vi "WriteAsyncErrorHandling.vi"(8 "ErrorIn":errorcluster, 10 "AsyncErrorHandling":T1, 11 "YActorIn":refnum<class "YActor.lvclass">) -> (0 "ErrorOut":errorcluster, 3 "YActorOut":refnum<class "YActor.lvclass">)   [LabVIEW 2021, in "YActor.lvclass"]
uses:
  YActor.lvclass
  AsyncErrorHandling.ctl
  YActor.lvclass/YActor.ctl
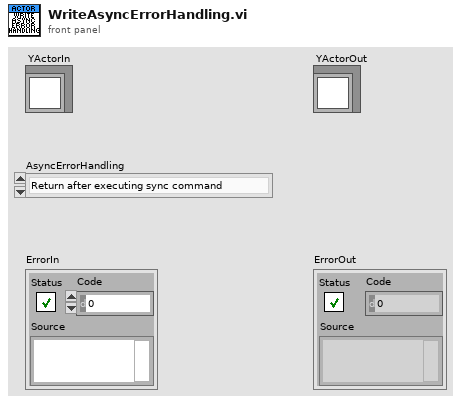
[diagram p1: front panel]
types:
  T1 = typedef "YActor.lvclass/AsyncErrorHandling.ctl" = enum16{"Return after executing sync command", "Return before executing sync command", "Don't return error"}
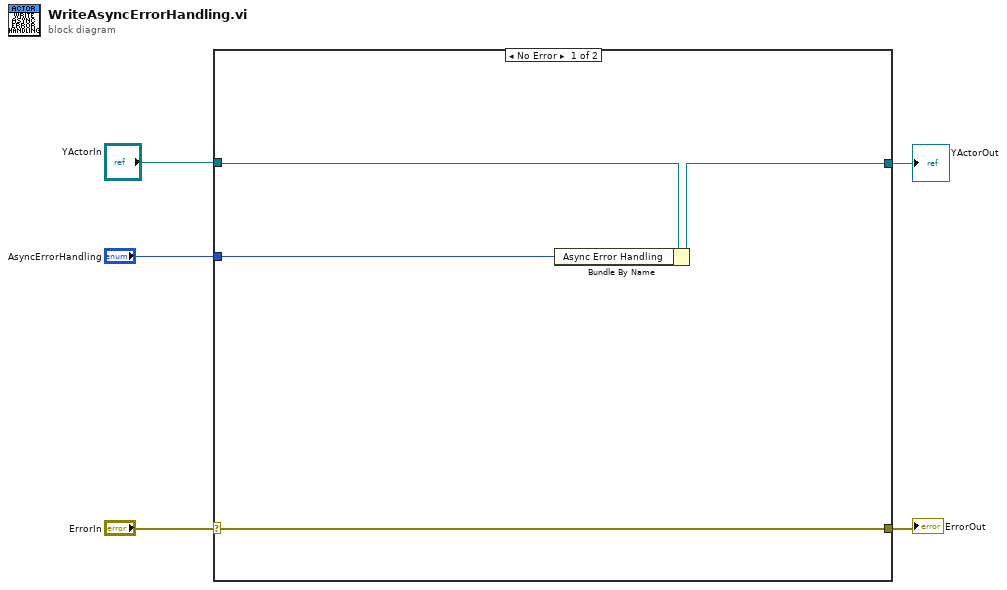
[diagram p0: block diagram]
diagram:
  n1 = case shown="No Error" "ErrorIn" {
    selector: "ErrorIn" -> [w9 w11]
    tunnel: [w9 w11] -> w4
    tunnel: [w6 w10] -> w2
    tunnel: "YActorIn" -> [w7 w10]
    tunnel: "AsyncErrorHandling" -> [w8 _]
    frame No Error {
      n2 = Bundle By Name(cluster=w7, "Async Error Handling"=w8) -> (w6:refnum<class "YActor.lvclass">)
    }
    frame Error {
    }
  }
  "ErrorOut" <- w4
  "YActorOut" <- w2
